vi "GM_host_db_logging.vi"() -> ()   [LabVIEW 2011]
uses:
  GM_host_db_log_vars.ctl
  <vilib>/addons/database/Connection.llb/Conn ObjectReference.ctl
  Output - Cluster gas.ctl
  gas_values.ctl
  <vilib>/Platform/TimedLoop/XDataNode/timing_clust.ctl
  <vilib>/Platform/TimedLoop/XDataNode/nitl_modes.ctl
  <vilib>/Platform/TimedLoop/XDataNode/wakeup.ctl
  <vilib>/Platform/TimedLoop/XDataNode/XDataNode.xnode
  <vilib>/Platform/TimedLoop/XDataNode/XDNodeRunTimeDep.lvlib
  <vilib>/addons/database/NI_Database_API.lvlib
  <userlib>/_JGCODE/error_logger/_error_logger.llb/ErrorLogger.lvclass
panel:
  out "target connection":bool
  out "db connection":bool
  in  "stop":bool caption="EXIT"
  in  "prefix for tables":string(combo)="GM"
  in  "interval [s]":u32=10 min=1 step=1
  in  "path":path
  # "GM DB Logging"
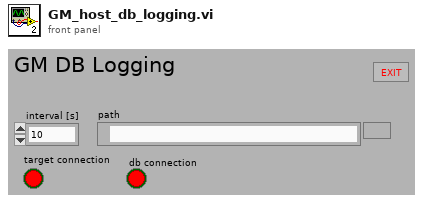
[diagram p1: front panel]
types:
  T1 = typedef "Output - Cluster gas.ctl" = cluster{"B2G2 MR V1.1 AUF":bool, "B2G2 MR V1.1 ZU":bool, "B2G2 MR V1 AUF":bool, "B2G2 MR V1 ZU":bool, "B2G1 T2 V1 AUF":bool, "B2G1 T2 V1 ZU":bool, "B2G1 T2 V1.1 AUF":bool, "B2G1 T2 V1.1 ZU":bool, "B2G2 T2 V1 AUF":bool, "B2G2 T2 V1 ZU":bool, "B2G2 T2 V1.1 ZU":bool, "B2G2 T2 V1.1 AUF":bool, "B2G1 MR V1 AUF":bool, "B2G1 MR V1 ZU":bool, "B2G1 MR V1.1 AUF":bool, "B2G1 MR V1.1 ZU":bool, "B2G1 HR V1 AUF":bool, "B2G1 HR V1 ZU":bool, "B2G1 HR V1.1 AUF":bool, "B2G1 HR V1.1 ZU":bool, "Fab1 HR V1 AUF":bool, "Fab1 HR V1 ZU":bool, "Fab1 HR V1.1 AUF":bool, "Fab1 HR V1.1 ZU":bool, "Fab1 MR V1 AUF":bool, "Fab1 MR V1 ZU":bool, "Fab1 MR V1.1 AUF":bool, "Fab1 MR V1.1 ZU":bool, "Fab1 BL V1 AUF":bool, "Fab1 BL V1 ZU":bool, "Fab1 BL V1.1 AUF":bool, "Fab1 BL V1.1 ZU":bool, "Fab2 HR V1 AUF":bool, "Fab2 HR V1 ZU":bool, "Fab2 HR V1.1 AUF":bool, "Fab2 HR V1.1 ZU":bool, "Fab2 MR V1 AUF":bool, "Fab2 MR V1 ZU":bool, "Fab2 MR V1.1 AUF":bool, "Fab2 MR V1.1 ZU":bool, "GA1 ch4 [%]":dbl, "GA1 co2 [%]":dbl, "GA1 h2 [%]":dbl, "GM P1 RUN":bool, "GM V-1 AUF":bool, "GM V-1 ZU":bool, "GM V-2 AUF":bool, "GM V-2 ZU":bool, "GM V-3 AUF":bool, "GM V-3 ZU":bool, "GM V-4 AUF":bool, "GM V-4 ZU":bool, "GM P2 RUN":bool, "GM GZ-1 [imp]":u32, "GM DS-2 [bar]":dbl, "GM DS-1 [bar]":dbl, "GM TS-1 [°C]":dbl, "GM TS-2[°C]":dbl, "gas_values":T2, "measuring mode":u8, "GM V-5":bool, "measuring volume":dbl, "automatic":bool, "GM MP manual V1.1 AUF":bool, "GM MP manual V1.1 ZU":bool}
  T2 = typedef "gas_values.ctl" = cluster{"start":timestamp, "GM DS-2 [bar]":dbl, "GA1 ch4 [%]":dbl, "GA1 co2 [%]":dbl, "GA1 h2 [%]":dbl, "GM DS-1 [bar]":dbl, "GM TS-1 [°C]":dbl, "GM TS-2 [°C]":dbl, "GM GZ-1 [l]":dbl, "measuring point":u8, "end":timestamp, "empty":bool, "GM GZ-1 [l] 2":dbl, "GM TS-1 [°C] 2":dbl, "GM DS-1 [bar] 2":dbl, "GM DS-2 [bar] 2":dbl, "empty 2":bool, "measuring mode":u8}
  T3 = typedef "GM_host_db_log_vars.ctl" = cluster{"file timing":i64, "db timing":i64, "GZ1":u32, "db reference":T4, "P2 RUN":bool, "P1 RUN":bool, "db logging":bool, "data refnum":refnum<k21>, "measmode":u32, "prefix":string, "output cluster reading time":timestamp, "V1":bool, "V2":bool, "V3":bool, "V4":bool, "gas_values.timestamp":timestamp, "automatic":bool, "db connection":bool}
  T4 = typedef "NI_Database_API.lvlib/Conn ObjectReference.ctl" = refnum<k1>
  T5 = typedef "XDNodeRunTimeDep.lvlib/timing_clust.ctl" = cluster{"Expected End [f-1]":u64, "Actual End [f-1]":u64, "Finished Late? [f-1]":bool, "Expected End [i-1]":u64, "Actual End [i-1]":u64, "Finished Late? [i-1]":bool, "Expected Start [i]":u64, "Actual Start [i]":u64, "Expected Start [f]":u64, "Actual Start [f]":u64, "Source Name":string, "Structure Name":string, "Period":i64, "Deadline":i64, "Offset":i64, "Start":i64, "Priority":i32, "Timeout":i32, "Mode":T6, "Wakeup Reason":T7, "Error":errorcluster, "Source Type":string, "Secondary Source Type":string, "Global End Time":u64, "Global Start Time":u64, "Frame Duration":u64, "Iteration Duration":u64, "Assigned CPU":i32, "I/O Scan Engine Mode":u32}
  T6 = typedef "XDNodeRunTimeDep.lvlib/nitl_modes.ctl" = enum32{"No Change", "Process missed periods, maintain original phase", "Discard missed periods, maintain original phase", "Process missed periods, ignore original phase", "Discard missed periods, ignore original phase"}
  T7 = typedef "XDNodeRunTimeDep.lvlib/wakeup.ctl" = enum32{"Normal", "Aborted", "Asynchronous wakeup", "Timing source error", "Timed loop error", "Timeout"}
  T8 = enum32{"invalid app kind", "Development System", "Run Time System", "Student Edition", "Embedded LabVIEW", "Evaluation", "Custom"}
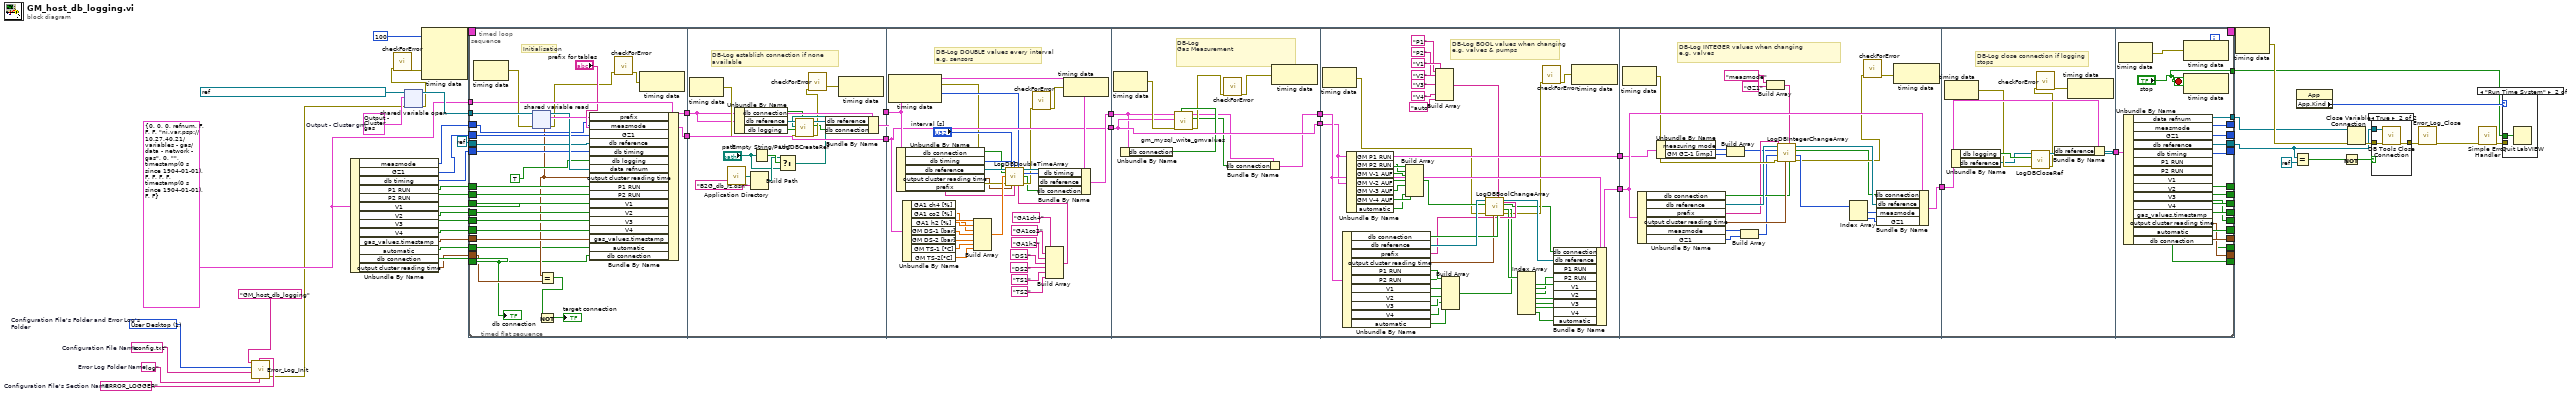
[diagram p0: block diagram]
diagram:
  w9 = "ERROR_LOGGER"  # Configuration File's Section Name
  w10 = "config.txt"  # Configuration File Name
  w11 = "log"  # Error Log Folder Name
  w12 = 1 items=["User Home", "User Desktop", "User Documents", "User Application Data", "User Preferences", "User Temporary", "Public Documents", "Public Application Data", "Public Preferences", "System Core Libraries", "System Installed Libraries", "Application Files", "Boot Volume Root"]  # Configuration File's Folder and Error Log's Folder
  w36 = T1 {"B2G2 MR V1.1 AUF"=FALSE, "B2G2 MR V1.1 ZU"=FALSE, "B2G2 MR V1 AUF"=FALSE, "B2G2 MR V1 ZU"=FALSE, "B2G1 T2 V1 AUF"=FALSE, "B2G1 T2 V1 ZU"=FALSE, "B2G1 T2 V1.1 AUF"=FALSE, "B2G1 T2 V1.1 ZU"=FALSE, "B2G2 T2 V1 AUF"=FALSE, "B2G2 T2 V1 ZU"=FALSE, "B2G2 T2 V1.1 ZU"=FALSE, "B2G2 T2 V1.1 AUF"=FALSE, "B2G1 MR V1 AUF"=FALSE, "B2G1 MR V1 ZU"=FALSE, "B2G1 MR V1.1 AUF"=FALSE, "B2G1 MR V1.1 ZU"=FALSE, "B2G1 HR V1 AUF"=FALSE, "B2G1 HR V1 ZU"=FALSE, "B2G1 HR V1.1 AUF"=FALSE, "B2G1 HR V1.1 ZU"=FALSE, "Fab1 HR V1 AUF"=FALSE, "Fab1 HR V1 ZU"=FALSE, "Fab1 HR V1.1 AUF"=FALSE, "Fab1 HR V1.1 ZU"=FALSE, "Fab1 MR V1 AUF"=FALSE, "Fab1 MR V1 ZU"=FALSE, "Fab1 MR V1.1 AUF"=FALSE, "Fab1 MR V1.1 ZU"=FALSE, "Fab1 BL V1 AUF"=FALSE, "Fab1 BL V1 ZU"=FALSE, "Fab1 BL V1.1 AUF"=FALSE, "Fab1 BL V1.1 ZU"=FALSE, "Fab2 HR V1 AUF"=FALSE, "Fab2 HR V1 ZU"=FALSE, "Fab2 HR V1.1 AUF"=FALSE, "Fab2 HR V1.1 ZU"=FALSE, "Fab2 MR V1 AUF"=FALSE, "Fab2 MR V1 ZU"=FALSE, "Fab2 MR V1.1 AUF"=FALSE, "Fab2 MR V1.1 ZU"=FALSE, "GA1 ch4 [%]"=0.0, "GA1 co2 [%]"=0.0, "GA1 h2 [%]"=0.0, "GM P1 RUN"=FALSE, "GM V-1 AUF"=FALSE, "GM V-1 ZU"=FALSE, "GM V-2 AUF"=FALSE, "GM V-2 ZU"=FALSE, "GM V-3 AUF"=FALSE, "GM V-3 ZU"=FALSE, "GM V-4 AUF"=FALSE, "GM V-4 ZU"=FALSE, "GM P2 RUN"=FALSE, "GM GZ-1 [imp]"=0, "GM DS-2 [bar]"=0.0, "GM DS-1 [bar]"=0.0, "GM TS-1 [°C]"=0.0, "GM TS-2[°C]"=0.0, "gas_values"={"start"=timestamp(0 s since 1904-01-01), "GM DS-2 [bar]"=0.0, "GA1 ch4 [%]"=0.0, "GA1 co2 [%]"=0.0, "GA1 h2 [%]"=0.0, "GM DS-1 [bar]"=0.0, "GM TS-1 [°C]"=0.0, "GM TS-2 [°C]"=0.0, "GM GZ-1 [l]"=0.0, "measuring point"=0, "end"=timestamp(0 s since 1904-01-01), "empty"=FALSE, "GM GZ-1 [l] 2"=0.0, "GM TS-1 [°C] 2"=0.0, "GM DS-1 [bar] 2"=0.0, "GM DS-2 [bar] 2"=0.0, "empty 2"=FALSE, "measuring mode"=0}, "measuring mode"=0, "GM V-5"=FALSE, "measuring volume"=0.0, "automatic"=FALSE, "GM MP manual V1.1 AUF"=FALSE, "GM MP manual V1.1 ZU"=FALSE}  # Output - Cluster gm
  w26 = T3 {"file timing"=0, "db timing"=0, "GZ1"=0, "db reference"=refnum, "P2 RUN"=FALSE, "P1 RUN"=FALSE, "db logging"=FALSE, "data refnum"="ni.var.psp://10.27.40.21/variables - gas/data - network - gas", "measmode"=0, "prefix"="", "output cluster reading time"=timestamp(0 s since 1904-01-01), "V1"=FALSE, "V2"=FALSE, "V3"=FALSE, "V4"=FALSE, "gas_values.timestamp"=timestamp(0 s since 1904-01-01), "automatic"=FALSE, "db connection"=FALSE} ("log vars")
  n1 = call "Error_Log_Init.vi"("Error Log Folder Name"=w11, "Configuration File's Section Name"=w9, "Configuration File Name"=w10, "Configuration File's Folder and Error Log's Folder"=w12, "Application Name (Application)"="GM_host_db_logging") -> ("error out"=w7:errorcluster)  [unwired: 6 in]
  n2 = Unbundle By Name(w26) -> ("measmode"=w21:u32, "GZ1"=w20:u32, "db timing"=w19:i64, "P1 RUN"=w25:bool, "P2 RUN"=w24:bool, "V1"=w23:bool, "V2"=w22:bool, "V3"=w18:bool, "V4"=w17:bool, "gas_values.timestamp"=w15:timestamp, "automatic"=w14:bool, "db connection"=w13:bool, "output cluster reading time"=w1:timestamp)
  n3 = shared-variable-open(refnum<k21> "ni.var.psp://10.27.40.21/variables - gm/data - network - gm" ("output variable"), w7, w36) -> (w37:refnum<k21>, w5:errorcluster)  [unwired: 1 in]
  n4 = call <userlib>:"checkForError.vi"("Error In"=w5) -> ("error out"=w6:errorcluster)  [unwired: 9 in, 1 out]
  n5 = node-c288(i64 100 ("Period"), w6) -> (w41:T5)  [unwired: 2 in]
  n6 = timed-loop {
    timing: w41 -> [_]
    timing-out: [_] -> w40
    shift-right: [w72] -> _
    shift-left: w19 -> [w73]
    tunnel: w26 -> [w71]
    shift-right: [w63] -> _
    shift-left: w20 -> [w68]
    shift-right: [w62] -> w29
    shift-left: refnum<k0> refnum -> [w70]
    tunnel: w37 -> [w69]
    shift-right: [w67] -> _
    shift-left: w25 -> [w66]
    shift-right: [w65] -> _
    shift-left: w22 -> [w64]
    tunnel: [w61] -> w27
    shift-right: [w60] -> _
    shift-left: w24 -> [w59]
    shift-right: [w58] -> _
    shift-left: w23 -> [w57]
    shift-right: [w56] -> _
    shift-left: w21 -> [w55]
    shift-right: [w54] -> _
    shift-left: w17 -> [w53]
    shift-right: [w52] -> _
    shift-left: w18 -> [w51]
    tunnel: [w50] -> w16
    shift-right: [w49] -> _
    shift-left: w15 -> [w48]
    shift-right: [w47] -> _
    shift-left: w1 -> [w46]
    shift-right: [w45] -> _
    shift-left: w14 -> [w44]
    shift-right: [w43] -> _
    shift-left: w13 -> [w42]
    stop <- "stop" stop-if-true
    n7 = timed-sequence {
      timing: _ -> [_]
      timing-out: _ -> [_]
      tunnel: w73 -> [w117]
      tunnel: [w116] -> w72
      tunnel: w71 -> [w115]
      tunnel: w70 -> [w114]
      tunnel: w69 -> [w109]
      tunnel: w68 -> [w108]
      tunnel: [w105] -> w67
      tunnel: w66 -> [w104]
      tunnel: [w103] -> w65
      tunnel: w64 -> [w102]
      tunnel: [w96] -> w63
      tunnel: [w95] -> w62
      tunnel: [w94] -> w61
      tunnel: [w93] -> w60
      tunnel: w59 -> [w92]
      tunnel: [w91] -> w58
      tunnel: w57 -> [w90]
      tunnel: [w89] -> w56
      tunnel: w55 -> [w88]
      tunnel: [w87] -> w54
      tunnel: w53 -> [w86]
      tunnel: [w85] -> w52
      tunnel: w51 -> [w84]
      tunnel: [w83] -> w50
      tunnel: [w82] -> w49
      tunnel: w48 -> [w81]
      tunnel: [w80] -> w47
      tunnel: w46 -> [w79]
      tunnel: [w78] -> w45
      tunnel: w44 -> [w77]
      tunnel: [w76] -> w43
      tunnel: w42 -> [w75]
      n8 = timed-flat-sequence {
        tunnel: w117 -> [w134]
        tunnel: [w142] -> w113
        tunnel: w115 -> [w136]
        tunnel: [w135] -> w111
        tunnel: w114 -> [w138]
        tunnel: w109 -> [w144]
        tunnel: w108 -> [w137]
        tunnel: w104 -> [w140]
        tunnel: w102 -> [w141]
        tunnel: w92 -> [w133]
        tunnel: w90 -> [w132]
        tunnel: w88 -> [w131]
        tunnel: w86 -> [w129]
        tunnel: w84 -> [w130]
        tunnel: w81 -> [w127]
        tunnel: w79 -> [w124]
        tunnel: w77 -> [w123]
        tunnel: w75 -> [w120]
        tunnel: w113 -> [w166]
        tunnel: [w166] -> w112
        tunnel: w111 -> [w163]
        tunnel: [w162] -> w110
        tunnel: w112 -> [w201]
        tunnel: [w201] -> w107
        tunnel: w110 -> [w202]
        tunnel: [w203] -> w106
        tunnel: w107 -> [w217]
        tunnel: [w217] -> w101
        tunnel: w106 -> [w216]
        tunnel: [w211] -> w100
        tunnel: w101 -> [w265]
        tunnel: w100 -> [w266]
        tunnel: [w267] -> w99
        tunnel: [w265] -> w97
        tunnel: w99 -> [w295]
        tunnel: [w296] -> w98
        tunnel: w97 -> [w278]
        tunnel: w98 -> [w308]
        tunnel: [w304] -> w74
        tunnel: [w326] -> w116
        tunnel: [w324] -> w105
        tunnel: [w321] -> w103
        tunnel: w74 -> [w331]
        tunnel: [w325] -> w96
        tunnel: [w327] -> w95
        tunnel: ["stop"] -> w94
        tunnel: [w323] -> w93
        tunnel: [w322] -> w91
        tunnel: [w328] -> w89
        tunnel: [w319] -> w87
        tunnel: [w320] -> w85
        tunnel: [w329] -> w83
        tunnel: [w318] -> w82
        tunnel: [w317] -> w80
        tunnel: [w316] -> w78
        tunnel: [w315] -> w76
        frame #0 {
          # "Initialisation"
          n9 = node-c288() -> (w143:errorcluster)  [unwired: 1 in]
          n10 = shared-variable-read(w144, w143) -> (w139:refnum<k21>, w122:errorcluster, w142:T1, w125:timestamp)
          n11 = Equal?(x=w125, y=w124) -> (x = y?=w119:bool)
          n12 = Not(x=w119) -> (.not. x?=→"target connection":bool)
          n13 = Bundle By Name(cluster=w136, "prefix"="prefix for tables", "measmode"=w131, "GZ1"=w137, "db reference"=w138, "db timing"=w134, "db logging"=TRUE ("on/off"), "data refnum"=w139, "output cluster reading time"=w125, "P1 RUN"=w140, "P2 RUN"=w133, "V1"=w132, "V2"=w141, "V3"=w130, "V4"=w129, "gas_values.timestamp"=w127, "automatic"=w123, "db connection"=w120) -> (w135:T3)
          n14 = call <userlib>:"checkForError.vi"("Error In"=w122) -> ("error out"=w121:errorcluster)  [unwired: 9 in, 1 out]
          n15 = node-c288(w121) -> ()  [unwired: 1 out]
          "db connection" <- w120
        }
        frame #1 {
          # "DB-Log establish connection if none available"
          n16 = node-c288() -> (w164:errorcluster)  [unwired: 1 in]
          n17 = call <vilib>:"Application Directory.vi"() -> ("Application Directory"=w157:path)
          n18 = Unbundle By Name(w163) -> ("db connection"=w151:bool, "db reference"=w165:T4, "db logging"=w160:bool)
          n19 = Build Path(base path=w157, name or relative path="B2G_db_rz.dsn" ("Name of ini file 2")) -> (appended path=w158:path)
          n20 = Empty String/Path?(string/path="path") -> (empty?=w159:bool)
          n21 = Select(t=w158, s=w159, f="path") -> (s? t:f=w155:path)
          n22 = call "LogDBCreateRef.vi"("db connection"=w151, "error in (no error)"=w164, "db"=w160, "Pfad in"=w155, "Refnum in"=w165) -> ("error out"=w152:errorcluster, "db connection"=w150:bool, "Refnum out"=w161:T4)  [unwired: 4 in]
          n23 = call <userlib>:"checkForError.vi"("Error In"=w152) -> ("error out"=w153:errorcluster)  [unwired: 9 in, 1 out]
          n24 = Bundle By Name(cluster=w163, "db reference"=w161, "db connection"=w150) -> (w162:T3)
          n25 = node-c288(w153) -> ()  [unwired: 1 out]
        }
        frame #2 {
          # "DB-Log DOUBLE values every interval\ne.g. sensors"
          n26 = node-c288() -> (w183:errorcluster, w198:i64)  [unwired: 1 in]
          n27 = Unbundle By Name(w202) -> ("db connection"=w194:bool, "db timing"=w199:i64, "db reference"=w195:T4, "output cluster reading time"=w182:timestamp, "prefix"=w181:string)
          n28 = Unbundle By Name(w201) -> ("GA1 ch4 [%]"=w185:dbl, "GA1 co2 [%]"=w180:dbl, "GA1 h2 [%]"=w179:dbl, "GM DS-1 [bar]"=w178:dbl, "GM DS-2 [bar]"=w177:dbl, "GM TS-1 [°C]"=w176:dbl, "GM TS-2[°C]"=w175:dbl)
          n29 = Build Array(w185, w180, w179, w178, w177, w176, w175) -> (w184:dbl[])
          n30 = Build Array("GA1ch4" ("table"), "GA1co2" ("table"), "GA1h2" ("table"), "DS1" ("table"), "DS2" ("table"), "TS1" ("table"), "TS2" ("table")) -> (w186:string[])
          n31 = call "LogDBDoubleTimeArray.vi"("Refnum in"=w195, "db Interval [s]"="interval [s]", "db timing"=w199, "Actual Start [f] in"=w198, "db connection"=w194, "values"=w184, "error in (no error)"=w183, "Time Stamp"=w182, "prefix"=w181, "names"=w186) -> ("Refnum out"=w196:T4, "Actual Start [f] out"=w197:i64, "db connection"=w172:bool, "error out"=w173:errorcluster)  [unwired: 2 in]
          n32 = call <userlib>:"checkForError.vi"("Error In"=w173) -> ("error out"=w174:errorcluster)  [unwired: 9 in, 1 out]
          n33 = Bundle By Name(cluster=w202, "db timing"=w197, "db reference"=w196, "db connection"=w172) -> (w203:T3)
          n34 = node-c288(w174) -> ()  [unwired: 1 out]
        }
        frame #3 {
          # "DB-Log\nGas Measurement"
          n35 = node-c288() -> (w218:errorcluster)  [unwired: 1 in]
          n36 = Unbundle By Name(w216) -> ("db connection"=w215:bool)
          n37 = call "gm_mysql_write_gmvalues.vi"("db connection"=w215, "error in (no error)"=w218, "Output - Cluster gm"=w217, "log vars in"=w216) -> ("error out"=w214:errorcluster, "db connection"=w210:bool, "log vars out"=w212:T3)  [unwired: 5 in]
          n38 = call <userlib>:"checkForError.vi"("Error In"=w214) -> ("error out"=w213:errorcluster)  [unwired: 9 in, 1 out]
          n39 = Bundle By Name(cluster=w212, "db connection"=w210) -> (w211:T3)
          n40 = node-c288(w213) -> ()  [unwired: 1 out]
        }
        frame #4 {
          # "DB-Log BOOL values when changing\ne.g. valves & pumps"
          n41 = node-c288() -> (w231:errorcluster)  [unwired: 1 in]
          n42 = Unbundle By Name(w266) -> ("db connection"=w256:bool, "db reference"=w257:T4, "prefix"=w254:string, "output cluster reading time"=w255:timestamp, "P1 RUN"=w245:bool, "P2 RUN"=w244:bool, "V1"=w243:bool, "V2"=w242:bool, "V3"=w241:bool, "V4"=w240:bool, "automatic"=w228:bool)
          n43 = Unbundle By Name(w265) -> ("GM P1 RUN"=w238:bool, "GM P2 RUN"=w237:bool, "GM V-1 AUF"=w236:bool, "GM V-2 AUF"=w235:bool, "GM V-3 AUF"=w234:bool, "GM V-4 AUF"=w233:bool, "automatic"=w227:bool)
          n44 = Build Array(w238, w237, w236, w235, w234, w233, w227) -> (w232:bool[])
          n45 = Build Array("P1" ("table"), "P2" ("table"), "V1" ("table"), "V2" ("table"), "V3" ("table"), "V4" ("table"), "auto" ("element")) -> (w258:string[])
          n46 = Build Array(w245, w244, w243, w242, w241, w240, w228) -> (w239:bool[])
          n47 = call "LogDBBoolChangeArray.vi"("db connection"=w256, "names"=w258, "cluster reading time"=w255, "prefix"=w254, "error in (no error)"=w231, "shift reg in"=w239, "values"=w232, "db reference"=w257) -> ("error out"=w225:errorcluster, "shift reg out"=w252:bool[], "db connection"=w224:bool, "db reference out"=w253:T4)
          n48 = Index Array(array=w252) -> (element #1=w251:bool, element #2=w250:bool, element #3=w249:bool, element #4=w248:bool, element #5=w247:bool, element #6=w246:bool, element #7=w229:bool)  [unwired: 7 in]
          n49 = call <userlib>:"checkForError.vi"("Error In"=w225) -> ("error out"=w226:errorcluster)  [unwired: 9 in, 1 out]
          n50 = Bundle By Name(cluster=w266, "db connection"=w224, "db reference"=w253, "P1 RUN"=w251, "P2 RUN"=w250, "V1"=w249, "V2"=w248, "V3"=w247, "V4"=w246, "automatic"=w229) -> (w267:T3)
          n51 = node-c288(w226) -> ()  [unwired: 1 out]
        }
        frame #5 {
          # "DB-Log INTEGER values when changing\ne.g. valves"
          n52 = node-c288() -> (w286:errorcluster)  [unwired: 1 in]
          n53 = Unbundle By Name(w295) -> ("db connection"=w282:bool, "db reference"=w284:T4, "prefix"=w277:string, "output cluster reading time"=w285:timestamp, "measmode"=w281:u32, "GZ1"=w280:u32)
          n54 = Unbundle By Name(w278) -> ("measuring mode"=w291:u8, "GM GZ-1 [imp]"=w290:u32)
          n55 = Build Array(w291, w290) -> (w276:u32[])
          n56 = Build Array(w281, w280) -> (w279:u32[])
          n57 = Build Array("measmode" ("table"), "GZ1" ("table")) -> (w292:string[])
          n58 = call "LogDBIntegerChangeArray.vi"("db connection"=w282, "names"=w292, "current time"=w285, "prefix"=w277, "error in (no error)"=w286, "shift reg in"=w279, "values"=w276, "Refnum in"=w284) -> ("error out"=w275:errorcluster, "shift reg out"=w287:u32[], "db connection"=w273:bool, "Refnum out"=w283:T4)
          n59 = Index Array(array=w287) -> (element #1=w289:u32, element #2=w288:u32)  [unwired: 2 in]
          n60 = call <userlib>:"checkForError.vi"("Error In"=w275) -> ("error out"=w274:errorcluster)  [unwired: 9 in, 1 out]
          n61 = Bundle By Name(cluster=w295, "db connection"=w273, "db reference"=w283, "measmode"=w289, "GZ1"=w288) -> (w296:T3)
          n62 = node-c288(w274) -> ()  [unwired: 1 out]
        }
        frame #6 {
          # "DB-Log close connection if logging stops"
          n63 = node-c288() -> (w306:errorcluster)  [unwired: 1 in]
          n64 = Unbundle By Name(w308) -> ("db logging"=w307:bool, "db reference"=w305:T4)
          n65 = call "LogDBCloseRef.vi"("error in (no error)"=w306, "enable"=w307, "Refnum in"=w305) -> ("error out"=w303:errorcluster, "Refnum out"=w309:T4)  [unwired: 7 in]
          n66 = call <userlib>:"checkForError.vi"("Error In"=w303) -> ("error out"=w302:errorcluster)  [unwired: 9 in, 1 out]
          n67 = Bundle By Name(cluster=w308, "db reference"=w309) -> (w304:T3)
          n68 = node-c288(w302) -> ()  [unwired: 1 out]
        }
        frame #7 {
          n69 = node-c288() -> (w332:errorcluster)  [unwired: 1 in]
          n70 = Unbundle By Name(w331) -> ("data refnum"=w329:refnum<k21>, "measmode"=w328:u32, "GZ1"=w325:u32, "db reference"=w327:T4, "db timing"=w326:i64, "P1 RUN"=w324:bool, "P2 RUN"=w323:bool, "V1"=w322:bool, "V2"=w321:bool, "V3"=w320:bool, "V4"=w319:bool, "gas_values.timestamp"=w318:timestamp, "output cluster reading time"=w317:timestamp, "automatic"=w316:bool, "db connection"=w315:bool)
          n71 = node-c288(w332) -> ()  [unwired: 1 out]
        }
      }
    }
    n72 = node-c288() -> ()  [unwired: 1 in, 1 out]
    n73 = node-c288() -> ()  [unwired: 1 in, 1 out]
  }
  n74 = node-c288(w40) -> (w28:errorcluster)
  n75 = Equal?(x=w29, y=refnum<k0> refnum) -> (x = y?=w34:bool)
  n76 = property class="App"() -> ("App.Kind"=w30:T8)  [unwired: 2 in, 2 out]
  n77 = Not(x=w34) -> (.not. x?=w32:bool)
  n78 = Close Variable Connection(8:w28, 11:w16) -> (0:w31:errorcluster)
  n79 = case shown="True" w32 {
    tunnel: w31 -> [w340 w343]
    tunnel: w29 -> [_ w342]
    tunnel: [w340 w341] -> w8
    frame False {
    }
    frame True {
      n80 = call <vilib>:"DB Tools Close Connection.vi"("error in (no error)"=w343, "connection reference"=w342) -> ("error out"=w341:errorcluster)  [unwired: 5 in]
    }
  }
  n81 = call "Error_Log_Close.vi"("error in (no error)"=w8) -> ("error out"=w3:errorcluster)  [unwired: 10 in]
  n82 = call <vilib>:"Simple Error Handler.vi"("error in (no error)"=w3) -> ("error out"=w2:errorcluster)  [unwired: 4 in, 4 out]
  n83 = case shown="\"Run Time System\"" w30 {
    tunnel: w27 -> [_ w344 _]
    tunnel: w2 -> [_ _ _]
    frame "invalid app kind", Default {
    }
    frame "Run Time System" {
      n84 = Quit LabVIEW(quit? (T)=w344) -> ()
    }
    frame "Development System" {
    }
  }
